vi "get_model.vi"(8 "error in (no error)":errorcluster, 11 "Modbus Master in":refnum<class "Modbus Master.lvclass">) -> (0 "error out":errorcluster, 2 "Model":string, 3 "Modbus Master out":refnum<class "Modbus Master.lvclass">)   [LabVIEW 2018, in "ICP xET-7017.lvlib"]
uses:
  <vilib>/NI/Modbus Library/API/Master/Modbus Master.lvclass
  ICP xET-7017.lvlib
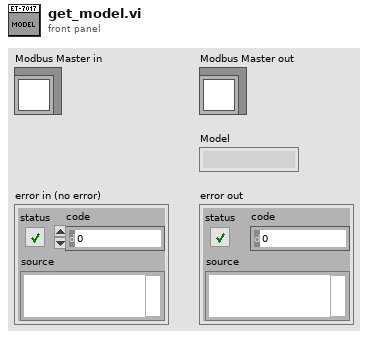
[diagram p1: front panel]
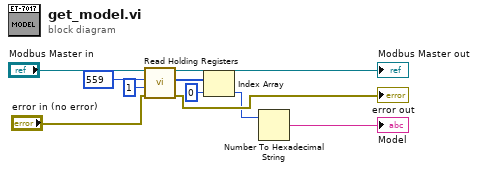
[diagram p0: block diagram]
diagram:
  n1 = call-dynamic "Read Holding Registers.vi"("error in"="error in (no error)", "number of inputs"=u16 1, "starting address"=u16 559, "Modbus master in"="Modbus Master in") -> ("error out"=→"error out":errorcluster, "register values"=w5:u16[], "Modbus master out"=→"Modbus Master out":refnum<class "Modbus Master.lvclass">)  [unwired: 5 in]
  n2 = Index Array(array=w5, index=0) -> (element=w1:u16)
  n3 = Number To Hexadecimal String(2:w1) -> (0:→"Model":string)  [unwired: 1 in]
